vi "Save Load State.vi"(6 "Instrument State Operation (0:Save)":u16(ring) items=["Save", "Load"], 7 "Storage To Use (0: State Storage)":u16(ring) items=["State Storage", "Mass Storage"], 8 "error in (no error)":errorcluster, 9 "Mass Storage Location (\"INT:\\state.sta\")":string="INT:\\state.sta", 10 "State Storage Location (1: 1)":u16(ring)=1 items=["1"=1, "2"=2, "3"=3, "4"=4], 11 "VISA resource name":refnum<visa-resource-name>) -> (0 "error out":errorcluster, 3 "VISA resource name out":refnum<visa-resource-name>)   [LabVIEW 2020, in "AWG.lvlib" / "Agilent 3352X Series.lvlib"]
doc: "Load instrument state stored in specified storage location or save state to specified location.\nThe <b>state</b> of instrument includes selected function (including arbitrary waveforms), frequency, amplitude, DC offset, duty cycle, symmetry, as well as any modulation parameters in use."
uses:
  Agilent 3352X Series.lvlib
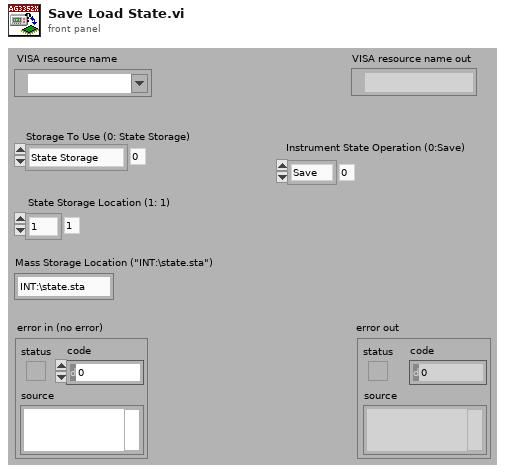
[diagram p1: front panel]
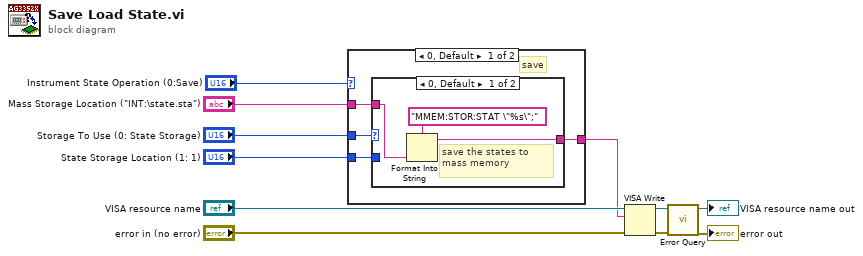
[diagram p0: block diagram]
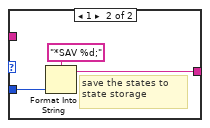
[diagram p2: hidden frame]
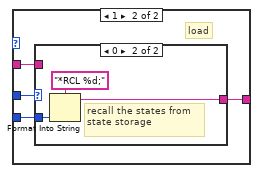
[diagram p3: hidden frame]
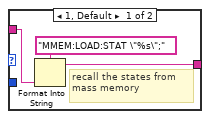
[diagram p4: hidden frame]
diagram:
  n1 = case shown="0, Default" "Instrument State Operation (0:Save)" {
    tunnel: "State Storage Location (1: 1)" -> [w13 w25]
    tunnel: "Storage To Use (0: State Storage)" -> [w14 w24]
    tunnel: [w12 w23] -> w3
    tunnel: "Mass Storage Location (\"INT:\\state.sta\")" -> [w15 w22]
    frame 0, Default {
      # "save"
      n2 = case shown="0, Default" w14 {
        tunnel: [w17 w20] -> w12
        tunnel: w13 -> [_ w19]
        tunnel: w15 -> [w16 _]
        frame 0, Default {
          # "save the states to mass memory"
          n3 = Format Into String(format string="MMEM:STOR:STAT \"%s\";", w16) -> (resulting string=w17:string)  [unwired: 2 in, 1 out]
        }
        frame 1 {
          # "save the states to state storage"
          n4 = Format Into String(format string="*SAV %d;", w19) -> (resulting string=w20:string)  [unwired: 2 in, 1 out]
        }
      }
    }
    frame 1 {
      # "load"
      n5 = case shown="0" w24 {
        tunnel: w25 -> [_ w30]
        tunnel: [w27 w29] -> w23
        tunnel: w22 -> [w26 _]
        frame 1, Default {
          # "recall the states from  mass memory"
          n6 = Format Into String(format string="MMEM:LOAD:STAT \"%s\";", w26) -> (resulting string=w27:string)  [unwired: 2 in, 1 out]
        }
        frame 0 {
          # "recall the states from  state storage"
          n7 = Format Into String(format string="*RCL %d;", w30) -> (resulting string=w29:string)  [unwired: 2 in, 1 out]
        }
      }
    }
  }
  n8 = VISA Write(VISA resource name="VISA resource name", write buffer=w3, error in (no error)="error in (no error)") -> (VISA resource name out=w8:refnum<visa-resource-name>, error out=w7:errorcluster)  [unwired: 1 out]
  n9 = call "Error Query.vi"("error in (no error)"=w7, "VISA resource name"=w8) -> ("error out"=→"error out":errorcluster, "VISA resource name out"=→"VISA resource name out":refnum<visa-resource-name>)  [unwired: 8 out]
